vi "FRCts20_WebMethods_Team_GET.vi"(7 "httpRequestID":u32, 10 "view":string, 11 "team":string) -> ()   [LabVIEW 2014, in "FRCts20_WebMethods.lvlib"]
doc: "<B>GET</B> on the specified <B>team</B> resource\n\nIf team is not specified, will return all resources. Teams can be filtered using the following parameters in the query string:\n - <B>division</B>\n - <B>competition</B>\n - <B>software</B> (unknown, LabVIEW, Windriver, C++, JavaBeans)\n - <B>status</B> (Open, In Work, Closed)\n\nhttp://<server address>:<port>/FRCts/team/<B>team</B>"
uses:
  FRCts20_WebMethods.lvlib
  Backend/source/VI Source/FRCts20_Backend_API/FRCts20_Backend_API.lvlib
  Backend/source/VI Source/FRCts20_Backend_API/FRCts20_Backend_API_Status.ctl
  Backend/source/VI Source/FRCts20_Backend_API/FRCts20_Backend_API_SW.ctl
  ESP Engine/source/VI Source/FRCts20_EspEngine.lvlib
  Backend/source/VI Source/FRCts20_Backend_API/FRCts20_Backend_API_Team.vi
  Backend/source/VI Source/FRCts20_Backend_API/FRCts20_Backend_API_Team.ctl
  Backend/source/VI Source/FRCts20_Backend_API/FRCts20_Backend_API_Command_Team.ctl
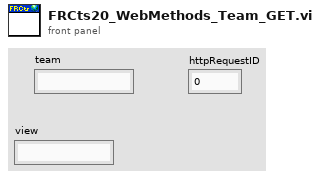
[diagram p1: front panel]
types:
  T1 = typedef "FRCts20_Backend_API.lvlib/FRCts20_Backend_API_Command_Team.ctl" = string
  T2 = typedef "FRCts20_Backend_API.lvlib/FRCts20_Backend_API_Team.ctl" = cluster{"Team Index":u32, "Team Number":u32, "Team Name":string, "Short Team Name":string, "Nick Name":string, "Robot Name":string, "City":string, "State":string, "Country":string, "Rookie Year":u32, "SWType":T3, "CAN":bool, "Vision":bool, "Kinect":bool, "Tags":string, "Avatar":string, "Request Array":cluster{"Request Index":u32, "Description":string, "Status":T4, "Open Date":timestamp, "Last Update":timestamp, "Close Date":timestamp}[], "Events Attending":cluster{"EventIndex":dbl, "EventName":string, "IsLive":bool}[], "APIReturn":string}
  T3 = typedef "FRCts20_Backend_API.lvlib/FRCts20_Backend_API_SW.ctl" = string
  T4 = typedef "FRCts20_Backend_API.lvlib/FRCts20_Backend_API_Status.ctl" = enum16{"Open", "In Work", "Closed"}
  T5 = typedef "FRCts20_EspEngine.lvlib/FRCts20_EspEngine_SearchBrowser.ctl" = cluster{"Event":cluster{"Event Index":u32, "Event Name":string, "Start Time":timestamp, "End Time":timestamp, "OpenIssues":u8, "IsLive":bool}[], "select-choice-software":string, "select-choice-location":string}
  T6 = typedef "FRCts20_EspEngine.lvlib/FRCts20_EspEngine_Team.ctl" = cluster{"Team":T7, "RequestListLength":i16, "Requests":T9[]}
  T7 = typedef "FRCts20_WebMethods.lvlib/FRCts20_WebMethods_ctl_singleTeam.ctl" = cluster{"Events":string[], "Robot Name":string, "Kinect":bool, "Vision":bool, "Can":bool, "Tags":string, "Avatar URL":string, "Team":T8, "SWType":T3}
  T8 = typedef "FRCts20_WebMethods.lvlib/FRCts20_WebMethods_ctl_teamIdentifier.ctl" = cluster{"Team Nickname":string, "Team Number ":u32, "UniqueId":u32}
  T9 = typedef "FRCts20_WebMethods.lvlib/FRCts20_WebMethods_ctl_request.ctl" = cluster{"Event":string, "Description":string, "Status":T4, "Open Date":string, "Last Update":string, "Close Date":string, "UniqueId":i32, "Team":cluster{"Team Nickname":string, "Team Number ":i32, "UniqueId":i32}, "Comments":cluster{"Request Number":dbl, "Text":string, "Author":string, "IsSolution":bool, "Team":cluster{"Team Nickname":string, "Team Identifier ":dbl}, "UniqueId":i32}[]}
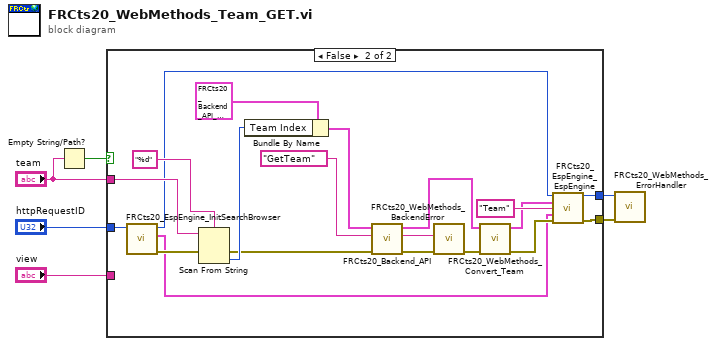
[diagram p0: block diagram]
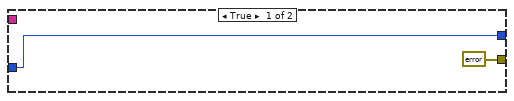
[diagram p2: hidden frame]
diagram:
  n1 = Empty String/Path?(string/path="team") -> (empty?=w2:bool)
  n2 = case shown="False" w2 {
    tunnel: "httpRequestID" -> [w7 w11]
    tunnel: "team" -> [_ w17]
    tunnel: [errorcluster {"status"=FALSE, "code"=0, "source"=""} ("error out") w26] -> w5
    tunnel: [w7 w25] -> w4
    tunnel: "view" -> [_ _]
    frame True {
    }
    frame False {
      n3 = call "FRCts20_EspEngine_InitSearchBrowser.vi"("httpRequestID"=w11) -> ("error out"=w12:errorcluster, "SearchBrowser"=w9:T5, "httpRequestID out"=w10:u32)  [unwired: 8 in]
      n4 = Scan From String(format string="%d", input string=w17, error in=w12) -> (error out=w13:errorcluster, output 1=w15:i32)  [unwired: 2 in, 2 out]
      n5 = Bundle By Name(cluster=T2 {"Team Index"=0, "Team Number"=0, "Team Name"="", "Short Team Name"="", "Nick Name"="", "Robot Name"="", "City"="", "State"="", "Country"="", "Rookie Year"=0, "SWType"="", "CAN"=FALSE, "Vision"=FALSE, "Kinect"=FALSE, "Tags"="", "Avatar"="", "Request Array"=[], "Events Attending"=[], "APIReturn"=""} ("Team Out"), "Team Index"=w15) -> (w14:T2)
      n6 = call-poly "FRCts20_Backend_API.vi"("error in (no error)"=w13, "Command"=T1 "GetTeam", "Team In"=w14) -> ("error out"=w28:errorcluster, "Status"=w27:string, "Team Out"=w20:T2)  [unwired: 6 in]
      n7 = call "FRCts20_WebMethods_BackendError.vi"("error in (no error)"=w28, "Status"=w27) -> ("error out"=w23:errorcluster)  [unwired: 8 in, 1 out]
      n8 = call "FRCts20_WebMethods_Convert_Team.vi"("error in (no error)"=w23, "Team Out"=w20) -> ("error out"=w22:errorcluster, "Team"=w19:T6)  [unwired: 8 in]
      n9 = call "FRCts20_EspEngine_EspEngine.vi"("httpRequestID"=w10, "Cluster"=w19, "Page"="Team", "SearchBrowser"=w9, "error in (no error)"=w22) -> ("httpRequestID out"=w25:u32, "error out"=w26:errorcluster)  [unwired: 9 in]
    }
  }
  n10 = call "FRCts20_WebMethods_ErrorHandler.vi"("error in"=w5, "httpRequestID"=w4) -> ()  [unwired: 9 in, 1 out]
